vi "Read Unit ID.vi"(8 "error in":errorcluster, 11 "Modbus instance in":refnum<class "Modbus API.lvclass">) -> (0 "error out":errorcluster, 2 "unit ID":u8, 3 "Modbus instance out":refnum<class "Modbus API.lvclass">)   [LabVIEW 2021]
doc: "Accessor VI for unit ID."
uses:
  Modbus API.lvclass/Modbus API.ctl
  Transmission Data Unit/Transmission Data Unit.lvclass
  Network Protocol/Network Protocol.lvclass
  Modbus API.lvclass
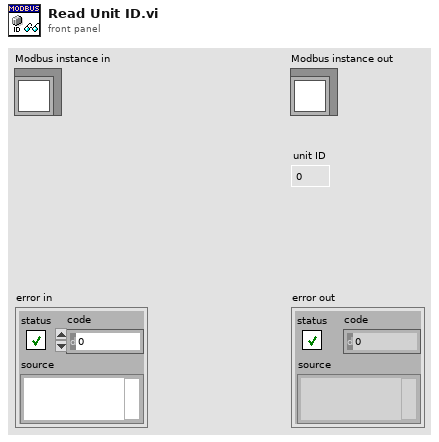
[diagram p1: front panel]
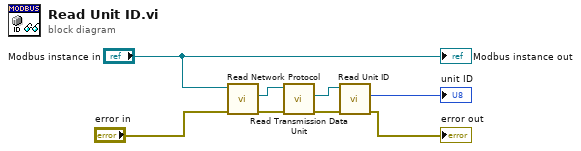
[diagram p0: block diagram]
diagram:
  n1 = call "Read Network Protocol.vi"("error in (no error)"="error in", "Modbus API in"="Modbus instance in") -> ("error out"=w5:errorcluster, "Network Protocol"=w4:refnum<class "Network Protocol.lvclass">)  [unwired: 7 in, 1 out]
  n2 = call "Read Transmission Data Unit.vi"("error in (no error)"=w5, "Network Protocol in"=w4) -> ("error out"=w3:errorcluster, "Transmission Data Unit"=w2:refnum<class "Transmission Data Unit.lvclass">)  [unwired: 7 in, 1 out]
  n3 = call "Read Unit ID.vi"("error in"=w3, "transmission data unit in"=w2) -> ("error out"=→"error out":errorcluster, "unit ID"=→"unit ID":u8)  [unwired: 7 in, 1 out]
  "Modbus instance out" <- "Modbus instance in"
